vi "Station Initial Status.vi"(9 "Status":bool, 10 "Insert":i32, 11 "Enum":T1) -> (2 "Array":bool[](array[boolean]), 3 "Read":bool)   [LabVIEW 2019]
uses:
  Ctrl/123.ctl
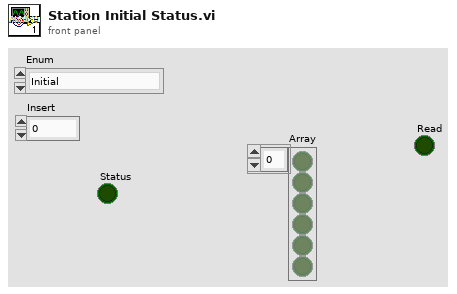
[diagram p1: front panel]
types:
  T1 = typedef "123.ctl" = enum16{"Initial", "Write", "Read"}
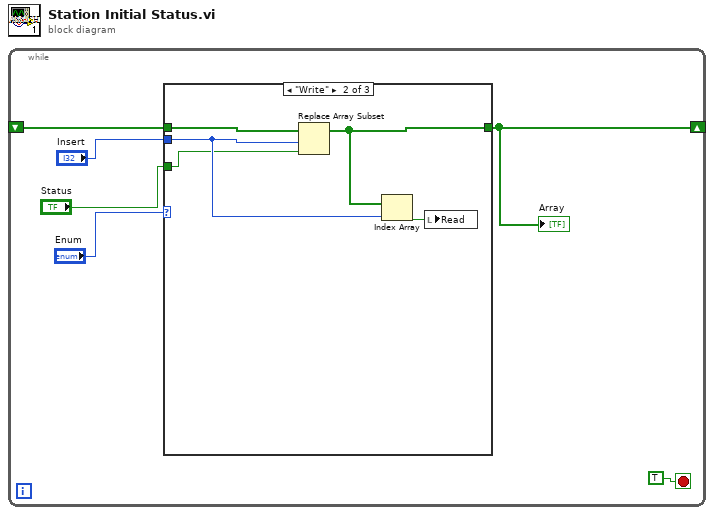
[diagram p0: block diagram]
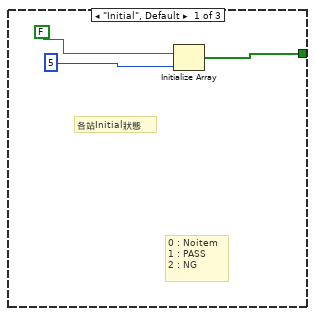
[diagram p2: hidden frame]
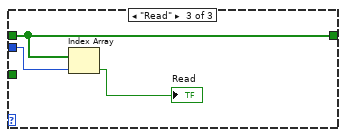
[diagram p3: hidden frame]
diagram:
  n1 = while {
    shift-right: [w2] -> _
    shift-left: _ -> [w5]
    stop <- TRUE stop-if-true
    n2 = case shown="\"Write\"" "Enum" {
      tunnel: w5 -> [_ w14 w17]
      tunnel: [w8 w12 w17] -> w2
      tunnel: "Insert" -> [_ w13 w16]
      tunnel: "Status" -> [_ w10 _]
      frame "Initial", Default {
        # "各站Initial狀態"
        # "0 : Noitem\n1 : PASS\n2 : NG"
        n3 = Initialize Array(FALSE, 5 ("dimension size")) -> (w8:bool[])
      }
      frame "Write" {
        n4 = Replace Array Subset "Replace Array Subset"(array=w14, new element=w10, index=w13) -> (w12:bool[])
        n5 = Index Array(array=w12, index=w13) -> (element=w11:bool)
        n6 = local write "Read"(w11) -> ()
      }
      frame "Read" {
        n7 = Index Array(array=w17, index=w16) -> (element=→"Read":bool)
      }
    }
    "Array" <- w2
  }
